vi "boot.vi"(8 "error in (no error)":errorcluster, 10 "asdf":string) -> (0 "error out":errorcluster)   [LabVIEW 2011]
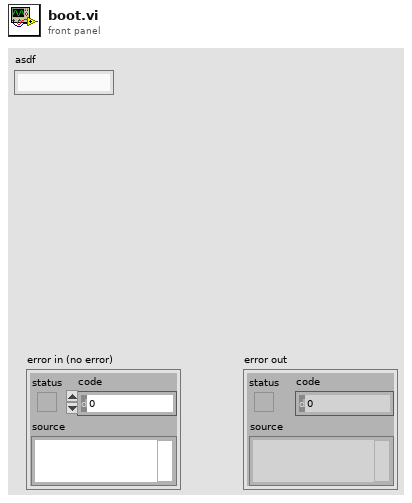
[diagram p1: front panel]
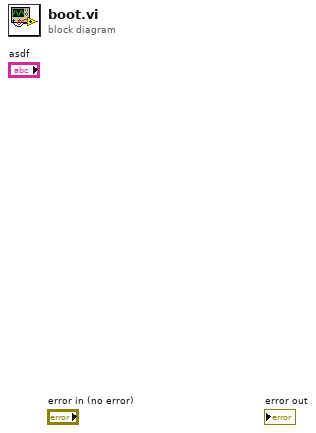
[diagram p0: block diagram]
diagram:
